vi "Keypad Password.vi"(6 "Password?":bool, 9 "String In":string) -> (1 "String Out":string)   [LabVIEW 2014]
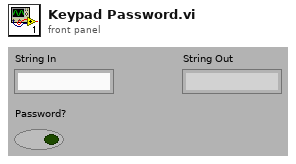
[diagram p1: front panel]
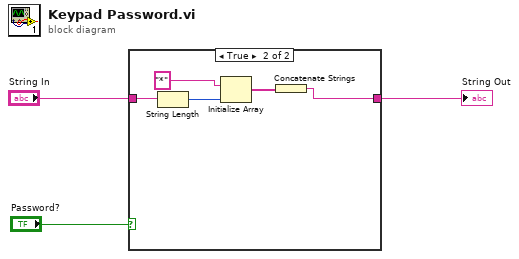
[diagram p0: block diagram]
diagram:
  n1 = case shown="True" "Password?" {
    tunnel: "String In" -> [w4 w9]
    tunnel: [w4 w5] -> w1
    frame False {
    }
    frame True {
      n2 = String Length(string=w9) -> (length=w8:i32)
      n3 = Initialize Array("*", w8) -> (w6:string[])
      n4 = Concatenate Strings(w6) -> (w5:string)
    }
  }
  "String Out" <- w1
